vi "4461 - Stop Tasks.vi"(8 "error in (no error)":errorcluster, 10 "AO task":refnum<k21>[](array[refnum]), 11 "AI task":refnum<k21>[](array[refnum])) -> (0 "error out":errorcluster)   [LabVIEW 2016]
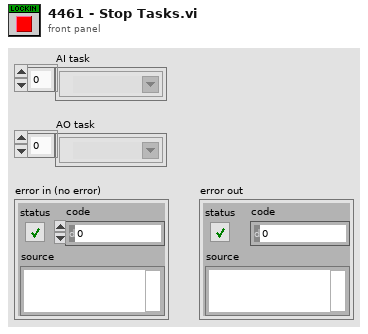
[diagram p1: front panel]
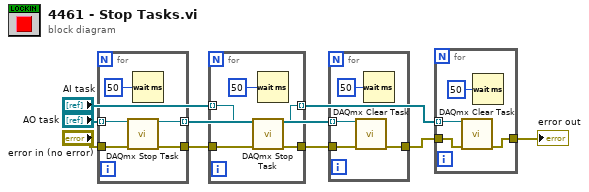
[diagram p0: block diagram]
diagram:
  n1 = for {
    tunnel: "AO task" -> [w14] mode=indexing
    tunnel: [w12] -> w1 mode=indexing
    tunnel: "error in (no error)" -> [w11]
    tunnel: [w10] -> w4
    n2 = call <vilib>:"DAQmx Stop Task.vi"("task/channels in"=w14, "error in"=w11) -> ("task out"=w12:refnum<k21>, "error out"=w10:errorcluster)  [unwired: 12 in]
    n3 = Wait (ms)(milliseconds to wait=u32 50) -> ()  [unwired: 1 out]
  }
  n4 = for {
    tunnel: "AI task" -> [w19] mode=indexing
    tunnel: [w17] -> w5 mode=indexing
    tunnel: w4 -> [w16]
    tunnel: [w15] -> w2
    n5 = call <vilib>:"DAQmx Stop Task.vi"("task/channels in"=w19, "error in"=w16) -> ("task out"=w17:refnum<k21>, "error out"=w15:errorcluster)  [unwired: 12 in]
    n6 = Wait (ms)(milliseconds to wait=u32 50) -> ()  [unwired: 1 out]
  }
  n7 = for {
    tunnel: w1 -> [w23] mode=indexing
    tunnel: w2 -> [w21]
    tunnel: [w20] -> w3
    n8 = call <vilib>:"DAQmx Clear Task.vi"("task in"=w23, "error in"=w21) -> ("error out"=w20:errorcluster)  [unwired: 13 in]
    n9 = Wait (ms)(milliseconds to wait=u32 50) -> ()  [unwired: 1 out]
  }
  n10 = for {
    tunnel: w5 -> [w27] mode=indexing
    tunnel: w3 -> [w25]
    tunnel: [w24] -> w6
    n11 = call <vilib>:"DAQmx Clear Task.vi"("task in"=w27, "error in"=w25) -> ("error out"=w24:errorcluster)  [unwired: 13 in]
    n12 = Wait (ms)(milliseconds to wait=u32 50) -> ()  [unwired: 1 out]
  }
  "error out" <- w6
